vi "write_pulse_1_ch per device_1.vi"(8 "error in":errorcluster, 9 "first call":bool, 11 "secnario config":T1={"devicess 2"=["IF_transiver_1", "IF_transiver_2"], "file paths"=[path "C:/Users/PXIe8108_Demo/Documents/CHAIM DATA/chaim/5785_sync_for_elbit/data/pdw_test_file.tdms", path "C:/Users/PXIe8108_Demo/Documents/CHAIM DATA/chaim/5785_sync_for_elbit/data/pdw_test_file.tdms", path "C:/Users/PXIe8108_Demo/Documents/CHAIM DATA/chaim/5785_sync_for_elbit/data/pdw_test_file.tdms", path "C:/Users/PXIe8108_Demo/Documents/CHAIM DATA/chaim/5785_sync_for_elbit/data/pdw_test_file.tdms"], "buffer size"=524288, "Fs  FPGA"=200000000.0, "SPC"=16.0, "center frequency (Hz) "=1000000000.0, "t clock ref"=[], "fpga rfe"=[], "tdms refs"=[], "niUsrpRio Session (out)"={"FPGA Interface"=refnum, "RIO Interface Number"=0, "Data Clock Rate"=0, "FPGA Data Clock Rate"=0, "Global Settings Register Bus"=refnum, "Radio 0 Settings Register Bus"=refnum, "Radio 1 Settings Register Bus"=refnum, "Radio Settings Bus Semaphore"=refnum, "DB Queues"=[], "Characterization Data Valid?"=FALSE, "EEPROM Header"={"Checksum"=0, "Product Code"=0, "Hardware Current Version"=0, "Hardware Oldest Compatible Version"=0, "EEPROM Map Current Version"=0, "EEPROM Map Oldest Compatible Version"=0, "User Password"="", "Pointer to Factory Header"=0, "Pointer to User Header"=0, "Recommended Interval"=0, "Number of Reserved Bytes"=9, "Number of Daughterboards"=0, "Daughterboard IDs"=[], "Daughterboard Serial Numbers"=[]}, "Device Data Header"={"Checksum"=0, "Number of Channels"=0, "Number of Gain Settings"=[], "Pointer to Characterization Data"=[], "Number of Reserved Bytes"=27, "Number of Frequencies"=[]}, "EEPROM Characterization Header"={"Checksum"=0, "Date"=timestamp(0 s since 1904-01-01), "Temperature"=0.0, "Misc. Info"="", "Pointer to Device Data Header"=0, "Number of Reserved Bytes"=28}, "Characterization Data"=[], "FPGA Current Version"=0, "FPGA Oldest Compatible Version"=0, "Fixed Logic Current Version"=0, "Fixed Logic Oldest Compatible Version"=0, "FPGA Radio Settings Bus Current Version"=0, "FPGA Radio Settings Bus Oldest Compatible Version"=0, "FPGA Board Config Current Version"=0, "FPGA Board Config Oldest Compatible Version"=0, "Daughterboard Clock Rate"=0, "daughterboard configuration session handles"=[]}, "RF gain "=10, "mode"=0, "vst_device"=[], "IQ_rare_p2p"=200000000.0, "stream sesion P2P"=[]} {"mode" scale=0.0..2.0; "RF gain" min=0 max=31 step=1; "niUsrpRio Session (out)"."Daughterboard Clock Rate" format="%#.3pHz"; "niUsrpRio Session (out)"."FPGA Data Clock Rate" format="%#.3pHz"; "niUsrpRio Session (out)"."Data Clock Rate" format="%#.3pHz"; "niUsrpRio Session (out)"."Characterization Data"."Frequencies [Hz]" format="%#_6p"; "niUsrpRio Session (out)"."EEPROM Characterization Header"."Pointer to Device Data Header" format="%x"; "niUsrpRio Session (out)"."EEPROM Characterization Header"."Checksum" format="%x"; "niUsrpRio Session (out)"."Device Data Header"."Pointer to Characterization Data" format="%x"; "niUsrpRio Session (out)"."Device Data Header"."Checksum" format="%x"; "niUsrpRio Session (out)"."EEPROM Header"."Pointer to User Header" format="%x"; "niUsrpRio Session (out)"."EEPROM Header"."Pointer to Factory Header" format="%x"; "niUsrpRio Session (out)"."EEPROM Header"."Product Code" format="%x"; "niUsrpRio Session (out)"."EEPROM Header"."Checksum" format="%x"; "center frequency (Hz)" format="%#.8p"; "buffer size" step=512}) -> (0 "error out":errorcluster, 1 "num of pulse sent to fpga":i32, 2 "done write files":bool, 3 "output cluster":T1={"devicess 2"=["IF_transiver_1", "IF_transiver_2"], "file paths"=[path "C:/Users/PXIe8108_Demo/Documents/CHAIM DATA/chaim/5785_sync_for_elbit/data/pdw_test_file.tdms", path "C:/Users/PXIe8108_Demo/Documents/CHAIM DATA/chaim/5785_sync_for_elbit/data/pdw_test_file.tdms", path "C:/Users/PXIe8108_Demo/Documents/CHAIM DATA/chaim/5785_sync_for_elbit/data/pdw_test_file.tdms", path "C:/Users/PXIe8108_Demo/Documents/CHAIM DATA/chaim/5785_sync_for_elbit/data/pdw_test_file.tdms"], "buffer size"=524288, "Fs  FPGA"=200000000.0, "SPC"=16.0, "center frequency (Hz) "=1000000000.0, "t clock ref"=[], "fpga rfe"=[], "tdms refs"=[], "niUsrpRio Session (out)"={"FPGA Interface"=refnum, "RIO Interface Number"=0, "Data Clock Rate"=0, "FPGA Data Clock Rate"=0, "Global Settings Register Bus"=refnum, "Radio 0 Settings Register Bus"=refnum, "Radio 1 Settings Register Bus"=refnum, "Radio Settings Bus Semaphore"=refnum, "DB Queues"=[], "Characterization Data Valid?"=FALSE, "EEPROM Header"={"Checksum"=0, "Product Code"=0, "Hardware Current Version"=0, "Hardware Oldest Compatible Version"=0, "EEPROM Map Current Version"=0, "EEPROM Map Oldest Compatible Version"=0, "User Password"="", "Pointer to Factory Header"=0, "Pointer to User Header"=0, "Recommended Interval"=0, "Number of Reserved Bytes"=9, "Number of Daughterboards"=0, "Daughterboard IDs"=[], "Daughterboard Serial Numbers"=[]}, "Device Data Header"={"Checksum"=0, "Number of Channels"=0, "Number of Gain Settings"=[], "Pointer to Characterization Data"=[], "Number of Reserved Bytes"=27, "Number of Frequencies"=[]}, "EEPROM Characterization Header"={"Checksum"=0, "Date"=timestamp(0 s since 1904-01-01), "Temperature"=0.0, "Misc. Info"="", "Pointer to Device Data Header"=0, "Number of Reserved Bytes"=28}, "Characterization Data"=[], "FPGA Current Version"=0, "FPGA Oldest Compatible Version"=0, "Fixed Logic Current Version"=0, "Fixed Logic Oldest Compatible Version"=0, "FPGA Radio Settings Bus Current Version"=0, "FPGA Radio Settings Bus Oldest Compatible Version"=0, "FPGA Board Config Current Version"=0, "FPGA Board Config Oldest Compatible Version"=0, "Daughterboard Clock Rate"=0, "daughterboard configuration session handles"=[]}, "RF gain "=10, "mode"=0, "vst_device"=[], "IQ_rare_p2p"=200000000.0, "stream sesion P2P"=[]} {"mode" scale=0.0..2.0; "RF gain" min=0 max=31 step=1; "niUsrpRio Session (out)"."Daughterboard Clock Rate" format="%#.3pHz"; "niUsrpRio Session (out)"."FPGA Data Clock Rate" format="%#.3pHz"; "niUsrpRio Session (out)"."Data Clock Rate" format="%#.3pHz"; "niUsrpRio Session (out)"."Characterization Data"."Frequencies [Hz]" format="%#_6p"; "niUsrpRio Session (out)"."EEPROM Characterization Header"."Pointer to Device Data Header" format="%x"; "niUsrpRio Session (out)"."EEPROM Characterization Header"."Checksum" format="%x"; "niUsrpRio Session (out)"."Device Data Header"."Pointer to Characterization Data" format="%x"; "niUsrpRio Session (out)"."Device Data Header"."Checksum" format="%x"; "niUsrpRio Session (out)"."EEPROM Header"."Pointer to User Header" format="%x"; "niUsrpRio Session (out)"."EEPROM Header"."Pointer to Factory Header" format="%x"; "niUsrpRio Session (out)"."EEPROM Header"."Product Code" format="%x"; "niUsrpRio Session (out)"."EEPROM Header"."Checksum" format="%x"; "center frequency (Hz)" format="%#.8p"; "buffer size" step=512}, 4 "room on the FIFO":bool)   [LabVIEW 2021]
uses:
  secnario config.ctl
  <vilib>/userdefined/High Color/nirio_resource_hc.ctl
  <instrlib>/niUsrpRio/Config/v1/Host/Public/niUsrpRio Session.ctl
  <instrlib>/_niInstr/Register Bus/v0/Host/Public/Register Bus Session.ctl
  <instrlib>/_niInstr/Register Bus/v0/Host/Private/Session Data.ctl
  <instrlib>/niUsrpRio/Config/v1/Host/Private/DB Queue Reference.ctl
  <instrlib>/niUsrpRio/Config/v1/Host/Private/Daughterboard Data.ctl
  <instrlib>/niUsrpRio/Config/v1/Host/Private/ATR state data.ctl
  <instrlib>/niUsrpRio/Config/v1/Host/Private/Antenna Configuration.ctl
  <instrlib>/niUsrpRio/Config/v1/Host/Private/CPLD Power Mode.ctl
  <instrlib>/niUsrpRio/Config/v1/Host/Public/EEPROM Header.ctl
  <instrlib>/niUsrpRio/Config/v1/Host/Public/EEPROM Device Data Header.ctl
  <instrlib>/niUsrpRio/Config/v1/Host/Public/EEPROM Characterization Header.ctl
  <instrlib>/niUsrpRio/Config/v1/Host/Public/Characterization Data.ctl
  <instrlib>/niUsrpRio/Config/v1/Host/Public/IQ Imbalance.ctl
  <vilib>/Utility/error.llb/Error Cluster From Error Code.vi
  <vilib>/rvi/errors/niLvFpgaAdjustHostInterfaceError.vi
  <vilib>/rvi/interface/nirviMethod/nirviMethod.xnode
  <vilib>/FPGAPlugInAG/Dynamic/niLvFpga_WriteFifo_Dynamic.vi
  <vilib>/rvi/errors/niLvFpgaMergeErrorWithErrorCode.vi
  <instrlib>/_niInstr/Register Bus/v0/Host/niInstr Register Bus v0 Host.lvlib
  <instrlib>/niUsrpRio/Config/v1/Host/niUsrpRio Config v1 Host.lvlib
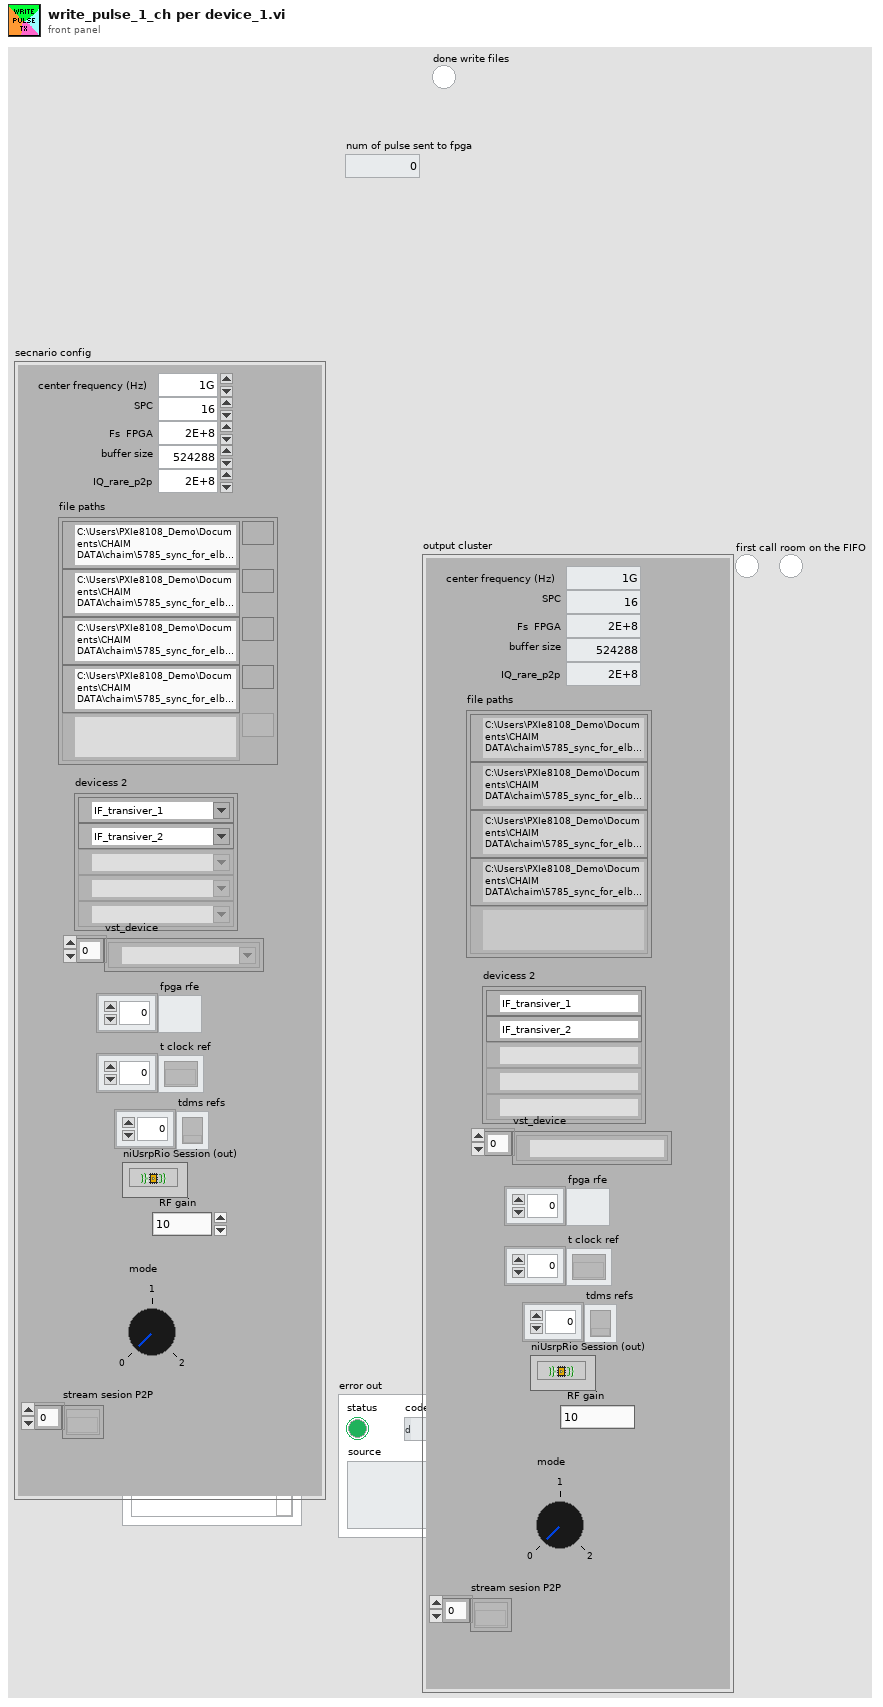
[diagram p1: front panel]
types:
  T1 = typedef "secnario config.ctl" = cluster{"devicess 2":T2[], "file paths":path[], "buffer size":u32, "Fs  FPGA":dbl, "SPC":dbl, "center frequency (Hz) ":dbl, "t clock ref":refnum<k20>[], "fpga rfe":refnum<k20>[], "tdms refs":refnum<k34>[], "niUsrpRio Session (out)":T3, "RF gain ":i32, "mode":u8, "vst_device":refnum<k15>[], "IQ_rare_p2p":dbl, "stream sesion P2P":refnum<k20>[]}
  T2 = typedef "nirio_resource_hc.ctl" = tag
  T3 = typedef "niUsrpRio Config v1 Host.lvlib/niUsrpRio Session.ctl" = cluster{"FPGA Interface":refnum<k20>, "RIO Interface Number":u32, "Data Clock Rate":u32, "FPGA Data Clock Rate":u32, "Global Settings Register Bus":T4, "Radio 0 Settings Register Bus":T4, "Radio 1 Settings Register Bus":T4, "Radio Settings Bus Semaphore":T5, "DB Queues":T6[], "Characterization Data Valid?":bool, "EEPROM Header":T7, "Device Data Header":T8, "EEPROM Characterization Header":T9, "Characterization Data":T10[], "FPGA Current Version":u32, "FPGA Oldest Compatible Version":u32, "Fixed Logic Current Version":u32, "Fixed Logic Oldest Compatible Version":u32, "FPGA Radio Settings Bus Current Version":u32, "FPGA Radio Settings Bus Oldest Compatible Version":u32, "FPGA Board Config Current Version":u32, "FPGA Board Config Oldest Compatible Version":u32, "Daughterboard Clock Rate":u32, "daughterboard configuration session handles":u64[]}
  T4 = typedef "niInstr Register Bus v0 Host.lvlib/Register Bus Session.ctl" = refnum<queue>
  T5 = typedef "Semaphore RefNum" = refnum<k1>
  T6 = typedef "niUsrpRio Config v1 Host.lvlib/DB Queue Reference.ctl" = refnum<queue>
  T7 = typedef "niUsrpRio Config v1 Host.lvlib/EEPROM Header.ctl" = cluster{"Checksum":u32, "Product Code":u16, "Hardware Current Version":u16, "Hardware Oldest Compatible Version":u16, "EEPROM Map Current Version":u16, "EEPROM Map Oldest Compatible Version":u16, "User Password":string, "Pointer to Factory Header":u32, "Pointer to User Header":u32, "Recommended Interval":u16, "Number of Reserved Bytes":i32, "Number of Daughterboards":u8, "Daughterboard IDs":u16[], "Daughterboard Serial Numbers":string[]}
  T8 = typedef "niUsrpRio Config v1 Host.lvlib/EEPROM Device Data Header.ctl" = cluster{"Checksum":u32, "Number of Channels":u8, "Number of Gain Settings":u16[], "Pointer to Characterization Data":u32[], "Number of Reserved Bytes":i32, "Number of Frequencies":u16[]}
  T9 = typedef "niUsrpRio Config v1 Host.lvlib/EEPROM Characterization Header.ctl" = cluster{"Checksum":u32, "Date":timestamp, "Temperature":sgl, "Misc. Info":string, "Pointer to Device Data Header":u32, "Number of Reserved Bytes":i32}
  T10 = typedef "niUsrpRio Config v1 Host.lvlib/Characterization Data.ctl" = cluster{"Gains[dB]":dbl[], "Frequencies [Hz]":dbl[], "IQ Imbalance Table":T11[], "Measured Gains[dB]":dbl[][]}
  T11 = typedef "niUsrpRio Config v1 Host.lvlib/IQ Imbalance.ctl" = cluster{"Gain Imbalance [linear]":dbl, "Phase Imbalance [radians]":dbl, "Offset":cdb}
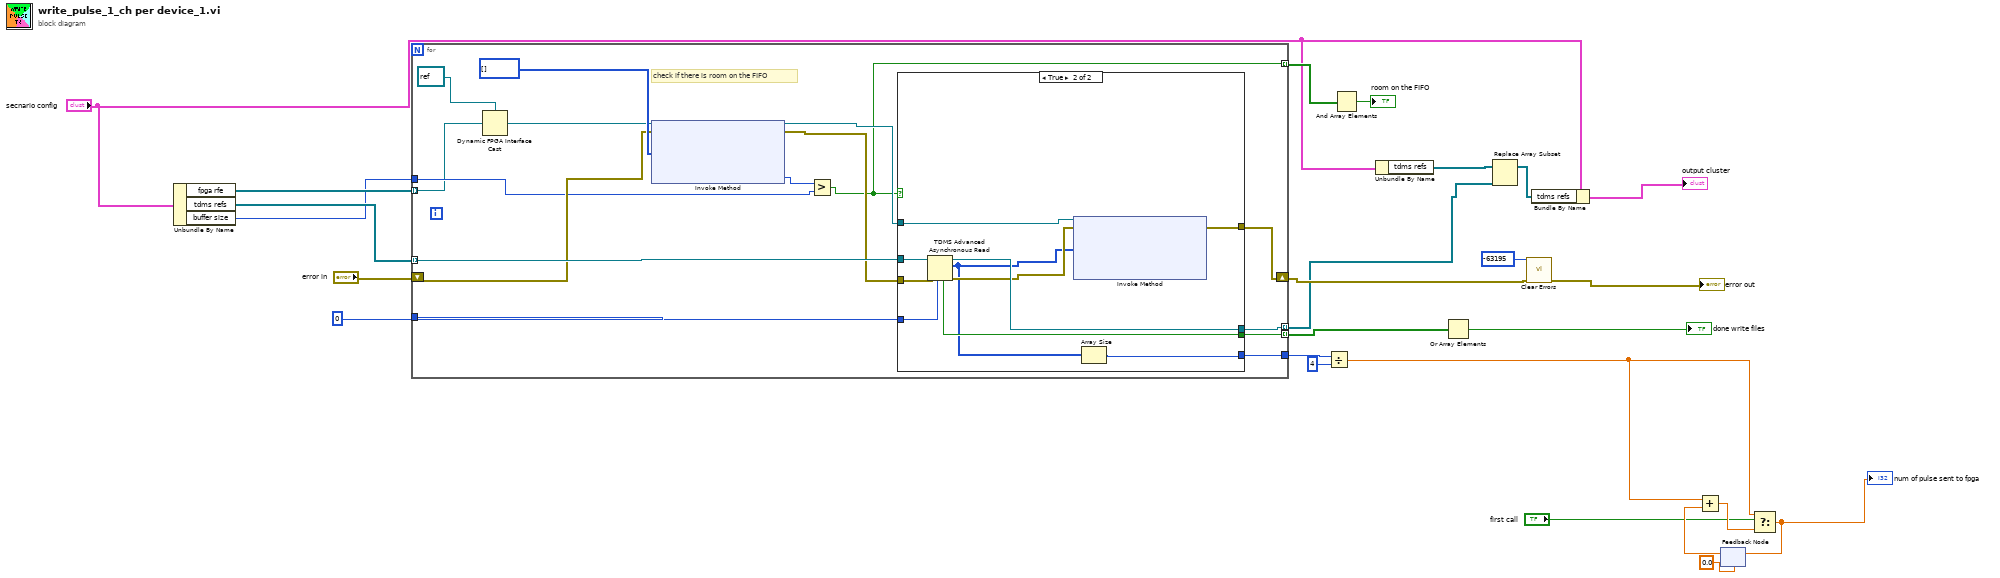
[diagram p0: block diagram]
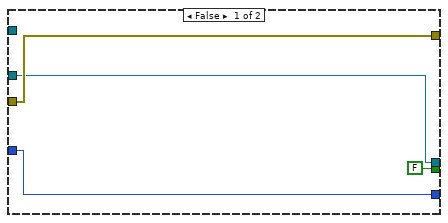
[diagram p2: hidden frame]
diagram:
  n1 = Unbundle By Name("secnario config") -> ("fpga rfe"=w12:refnum<k20>[], "tdms refs"=w11:refnum<k34>[], "buffer size"=w8:u32)
  n2 = for {
    tunnel: w11 -> [w41] mode=indexing
    tunnel: w12 -> [w28] mode=indexing
    tunnel: u64 0 ("type") -> [w40]
    tunnel: [w39] -> w13 mode=indexing
    tunnel: [w38] -> w2 mode=indexing
    shift-right: [w37] -> w9
    shift-left: "error in" -> [w34]
    tunnel: [w36] -> w15
    tunnel: w8 -> [w33]
    tunnel: [w30] -> w6 mode=indexing
    # "check if there is room on the FIFO"
    n3 = Dynamic FPGA Interface Cast(Session In=refnum<k20> refnum ("FPGA VI Reference Out"), Type=w28) -> (Session Out=w27:refnum<k20>)
    n4 = xnode "Invoke Method"("FPGA VI Reference In"=w27, "error in"=w34, "Data"=u64[] []) -> ("FPGA VI Reference Out"=w31:refnum<k20>, "error out"=w32:errorcluster, "Empty Elements Remaining"=w29:u32)  [unwired: 1 in]
    n5 = Greater?(x=w29, y=w33) -> (0:w30:bool)
    n6 = case shown="True" w30 {
      tunnel: w41 -> [w43 w55]
      tunnel: w40 -> [w45 w54]
      tunnel: [FALSE ("read process finished?") w53] -> w39
      tunnel: [w43 w52] -> w38
      tunnel: [w44 w50] -> w37
      tunnel: [w45 w48] -> w36
      tunnel: w32 -> [w44 w47]
      tunnel: w31 -> [_ w46]
      frame False {
      }
      frame True {
        n7 = TDMS Advanced Asynchronous Read(6:w54, 8:w47, 11:w55) -> (0:w51:errorcluster, 2:w49:u64[], 3:w52:refnum<k34>, 4:w53:bool)
        n8 = xnode "Invoke Method"("FPGA VI Reference In"=w46, "error in"=w51, "Data"=w49) -> ("error out"=w50:errorcluster)  [unwired: 1 in, 2 out]
        n9 = Array Size(array=w49) -> (size(s)=w48:i32)
      }
    }
  }
  n10 = Divide(x=w15, y=4) -> (x/y=w20:dbl)
  n11 = And Array Elements(Boolean array=w6) -> (logical AND=→"room on the FIFO":bool)
  n12 = Unbundle By Name("secnario config") -> ("tdms refs"=w3:refnum<k34>[])
  n13 = Or Array Elements(Boolean array=w13) -> (logical OR=→"done write files":bool)
  n14 = Replace Array Subset(array=w3, new element=w2) -> (w1:refnum<k34>[])  [unwired: 1 in]
  n15 = call <vilib>:"Clear Errors.vi"("error in (no error)"=w9, "specific error code to clear (0: all)"=-63195) -> ("error out"=→"error out":errorcluster)  [unwired: 4 in, 1 out]
  n16 = Bundle By Name(cluster="secnario config", "tdms refs"=w1) -> (→"output cluster":T1)
  n17 = feedback #1(0.0) -> (w21:dbl)
  n18 = Add(x=w20, y=w21) -> (x+y=w22:dbl)
  n19 = Select(t=w20, s="first call", f=w22) -> (s? t:f=w18:dbl)
  "num of pulse sent to fpga" <- w18
  n20 = feedback-in #1(w18) -> ()
